vi "Check DC_1.vi"(0 "NXT":T2, 2 "DC Motors":cluster{"DC Motor":T1, "Address":i16}={"DC Motor"=enum."DC Motor", "Address"=-1}) -> (4 "NXT":T2, 6 "Position 1":i32, 8 "Moving 1":bool)   [LabVIEW 2012, in "4134Outputs.lvlib"]
uses:
  4134Outputs.lvlib
  <vilib>/NXT/Subs/LVHSConnector.ctl
  <vilib>/NXT/LegoClasses/BrickReference/BrickReference.lvclass
  <vilib>/NXT/Subs/MotorXNode.DC Motor Type.ctl
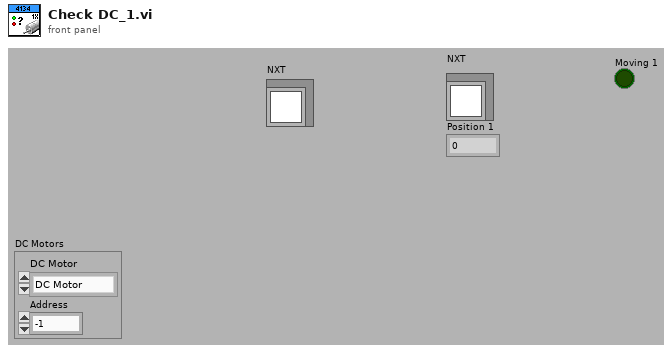
[diagram p1: front panel]
types:
  T1 = typedef "MotorXNode.DC Motor Type.ctl" = enum16{"DC Motor"}
  T2 = typedef "LVHSConnector.ctl" = refnum<class "BrickReference.lvclass">
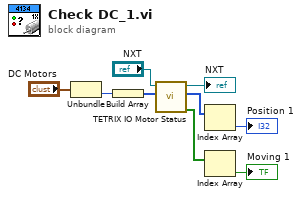
[diagram p0: block diagram]
diagram:
  n1 = Unbundle("DC Motors") -> ("Address"=w9:i16)  [unwired: 1 out]
  n2 = Build Array(w9) -> (w7:i16[])
  n3 = call <vilib>:"TETRIX IO Motor Status.vi"("DC Motors"=w7, "NXT"="NXT") -> ("Moves in Progress?"=w3:bool[], "Absolute Motor Positions"=w4:i32[], "NXT"=→"NXT":T2)  [unwired: 7 in]
  n4 = Index Array(array=w4) -> (element=→"Position 1":i32)  [unwired: 1 in]
  n5 = Index Array(array=w3) -> (element=→"Moving 1":bool)  [unwired: 1 in]
